vi "Calibrate.vi"(8 "error in (no error)":errorcluster, 11 "Message Queue":refnum<queue>) -> (0 "error out":errorcluster)   [LabVIEW 2020, in "plugin_flodx_pressure.lvlib" / "plugin.lvlib"]
doc: "UI which prompts the user to calibrate the device, in two-point and three-point modes."
uses:
  plugin.lvlib
  <userlib>/RxnRover/PluginCore/src/support/Message Queue/Message Cluster.ctl
  <userlib>/RxnRover/PluginCore/src/support/Message Queue/Message Queue.lvlib
panel:
  in  "Set Ambient Pressure":bool
  in  "Set Ambient Pressure":sgl
  in  "Units":string(combo)
  in  "SHUTDOWN":bool
  in  "Calibrate Button":bool
  # "Device Options"
  # "These are the device options for\nthe FloDx Pressure Sensor. You can\nset the units the device returns,\n(kPa,PSI,BAR) as well as set the\nambient pressure of the device."
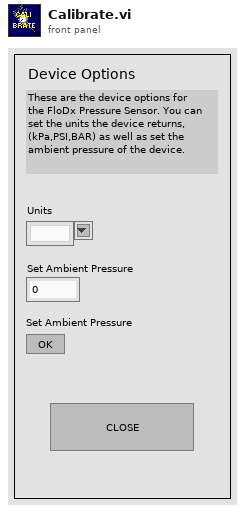
[diagram p1: front panel]
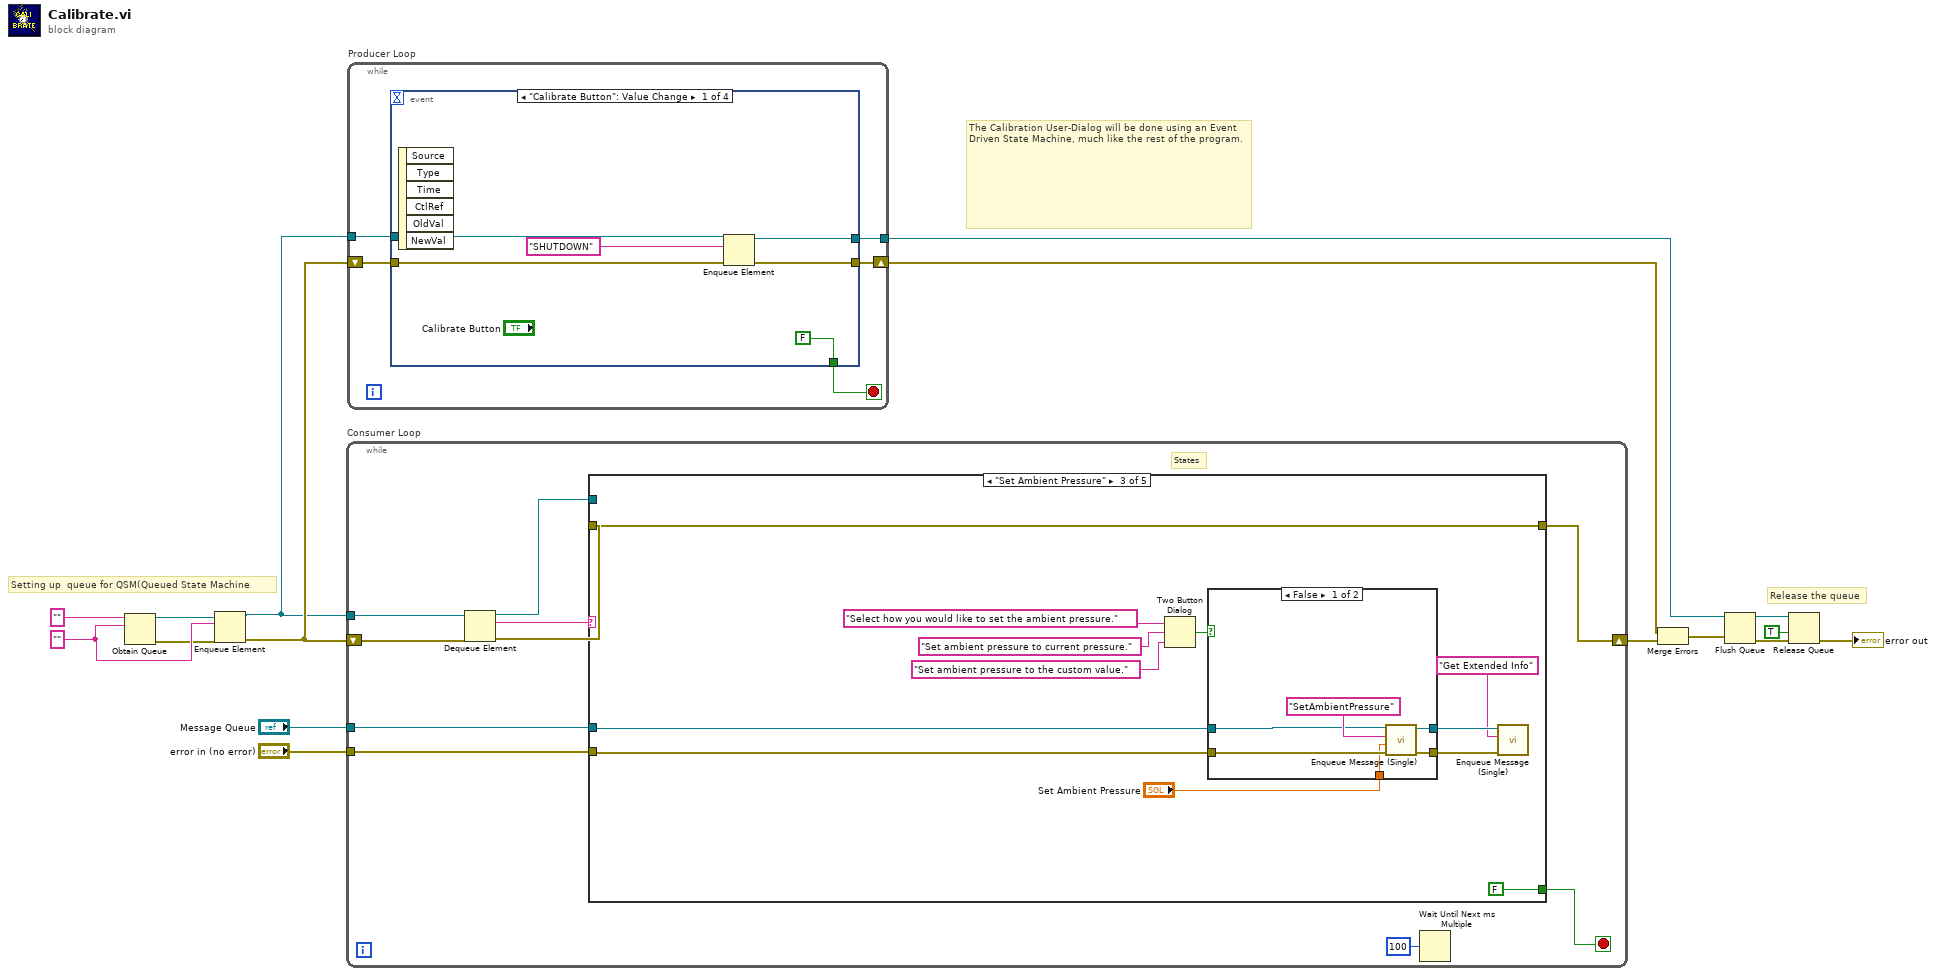
[diagram p0: block diagram]
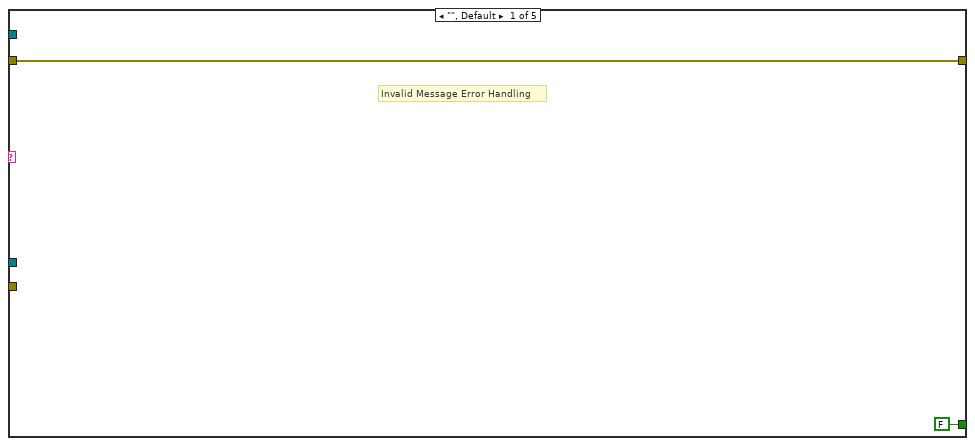
[diagram p2: hidden frame]
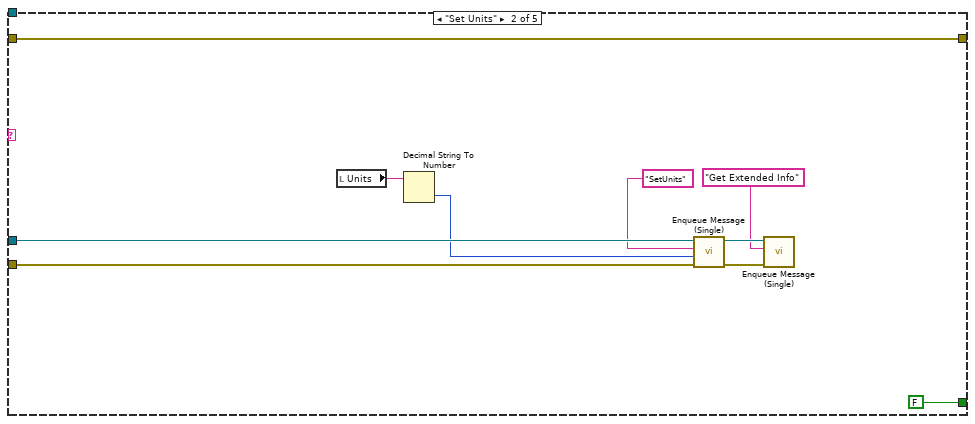
[diagram p3: hidden frame]
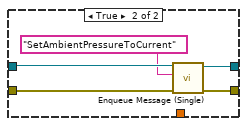
[diagram p4: hidden frame]
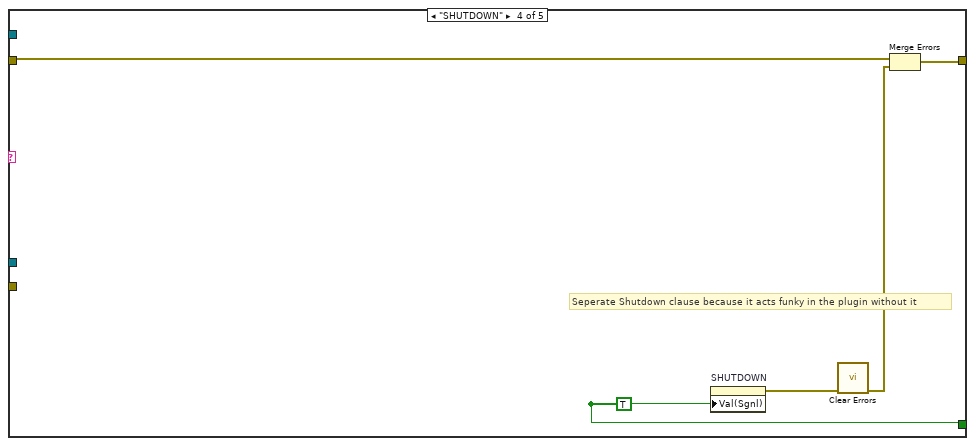
[diagram p5: hidden frame]
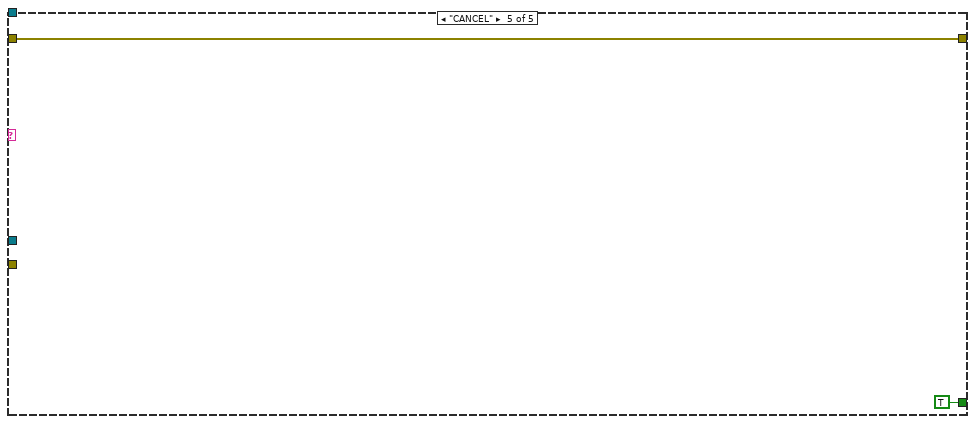
[diagram p6: hidden frame]
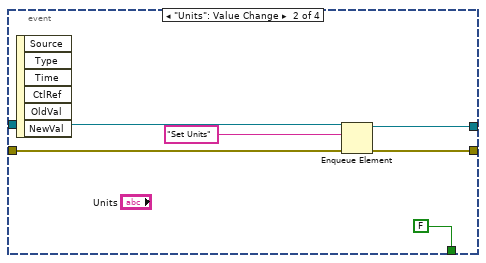
[diagram p7: hidden frame]
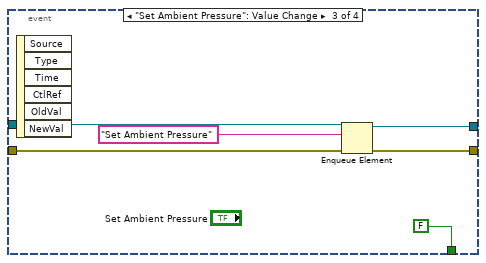
[diagram p8: hidden frame]
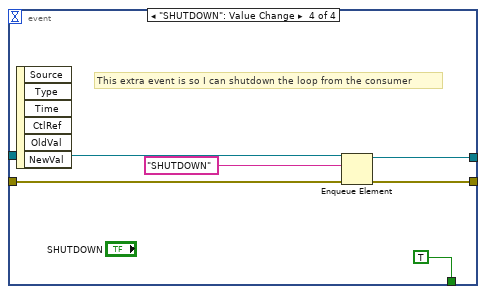
[diagram p9: hidden frame]
diagram:
  w15 = ""
  # "The Calibration User-Dialog will be done using an Event Driven State Machine, much like the rest of the program."
  # "Release the queue"
  # "Setting up  queue for QSM(Queued State Machine"
  n1 = Obtain Queue(name (unnamed)="", element data type=w15) -> (queue out=w14:refnum<queue>, error out=w13:errorcluster)  [unwired: 3 in, 1 out]
  n2 = Enqueue Element(queue=w14, element=w15, error in (no error)=w13) -> (queue out=w1:refnum<queue>, error out=w12:errorcluster)  [unwired: 1 in, 1 out]
  n3 = while "Consumer Loop" {
    tunnel: w1 -> [w26]
    tunnel: "Message Queue" -> [w21]
    tunnel: "error in (no error)" -> [w20]
    shift-right: [w18] -> w9
    shift-left: w12 -> [w17]
    stop <- w22 stop-if-true
    # "States"
    n4 = Dequeue Element(queue=w26, error in (no error)=w17) -> (queue out=w24:refnum<queue>, element=w25:string, error out=w23:errorcluster)  [unwired: 1 in, 1 out]
    n5 = case shown="\"Set Ambient Pressure\"" w25 {
      tunnel: w24 -> [_ _ _ _ _]
      tunnel: w23 -> [w27 w30 w42 w65 w67]
      tunnel: [FALSE ("T button?") FALSE ("T button?") FALSE ("T button?") w62 TRUE ("T button?")] -> w22
      tunnel: w21 -> [_ w37 w44 _ _]
      tunnel: w20 -> [_ w36 w45 _ _]
      tunnel: [w27 w30 w42 w66 w67] -> w18
      frame "", Default {
        # "Invalid Message Error Handling"
      }
      frame "Set Units" {
        n6 = local read "Units"() -> (w29:string)
        n7 = Decimal String To Number(string=w29) -> (number=w34:i32)  [unwired: 2 in, 1 out]
        n8 = call <userlib>:"Enqueue Message (Single).vi"("error in (no error)"=w36, "Message Data"=w34, "Message"="SetUnits", "Message Queue"=w37) -> ("error out"=w32:errorcluster, "dup Message Queue"=w33:refnum<queue>)  [unwired: 6 in]
        n9 = call <userlib>:"Enqueue Message (Single).vi"("error in (no error)"=w32, "Message"="Get Extended Info", "Message Queue"=w33) -> ()  [unwired: 7 in, 2 out]
      }
      frame "Set Ambient Pressure" {
        n10 = Two Button Dialog(message="Select how you would like to set the ambient pressure.", 1:"Set ambient pressure to the custom value." ("F button name (\"Cancel\")"), 2:"Set ambient pressure to current pressure." ("T button name (\"OK\")")) -> (T button?=w48:bool)
        n11 = case shown="False" w48 {
          tunnel: w45 -> [w54 w61]
          tunnel: w44 -> [w55 w60]
          tunnel: "Set Ambient Pressure" -> [w53 _]
          tunnel: [w51 w58] -> w41
          tunnel: [w52 w57] -> w40
          frame False {
            n12 = call <userlib>:"Enqueue Message (Single).vi"("error in (no error)"=w54, "Message Data"=w53, "Message"="SetAmbientPressure", "Message Queue"=w55) -> ("error out"=w51:errorcluster, "dup Message Queue"=w52:refnum<queue>)  [unwired: 6 in]
          }
          frame True {
            n13 = call <userlib>:"Enqueue Message (Single).vi"("error in (no error)"=w61, "Message"="SetAmbientPressureToCurrent", "Message Queue"=w60) -> ("error out"=w58:errorcluster, "dup Message Queue"=w57:refnum<queue>)  [unwired: 7 in]
          }
        }
        n14 = call <userlib>:"Enqueue Message (Single).vi"("error in (no error)"=w41, "Message"="Get Extended Info", "Message Queue"=w40) -> ()  [unwired: 7 in, 2 out]
      }
      frame "SHUTDOWN" {
        w62 = TRUE
        # "Seperate Shutdown clause because it acts funky in the plugin without it"
        n15 = property on="SHUTDOWN" class="Bool (strict)"("Val(Sgnl)"=w62) -> (error out=w63:errorcluster)  [unwired: 2 in, 1 out]
        n16 = call <vilib>:"Clear Errors.vi"("error in (no error)"=w63) -> ("error out"=w64:errorcluster)  [unwired: 5 in, 1 out]
        n17 = Merge Errors(w65, w64) -> (w66:errorcluster)
      }
      frame "CANCEL" {
      }
    }
    n18 = Wait Until Next ms Multiple(millisecond multiple=u32 100) -> ()  [unwired: 1 out]
  }
  n19 = while "Producer Loop" {
    tunnel: w1 -> [w72]
    shift-right: [w70] -> w8
    shift-left: w12 -> [w73]
    tunnel: [w69] -> w6
    stop <- w71 stop-if-true
    n20 = event shown="[0] \"Calibrate Button\": Value Change" {
      selector: _ -> [_ _ _ _]
      dyn-events: _ -> [_ _ _ _]
      timeout: _ -> [_ _ _ _]
      tunnel: w73 -> [w79 w85 w91 w97]
      tunnel: w72 -> [w78 w84 w90 w96]
      tunnel: [w77 w83 w89 w95] -> w69
      tunnel: [FALSE FALSE FALSE TRUE] -> w71
      tunnel: [w74 w80 w86 w92] -> w70
      event "Calibrate Button": Value Change {
        n21 = event-data() -> ()  [unwired: 1 in, 6 out]
        n22 = Enqueue Element(queue=w78, element="SHUTDOWN", error in (no error)=w79) -> (queue out=w77:refnum<queue>, error out=w74:errorcluster)  [unwired: 1 in, 1 out]
      }
      event "Units": Value Change {
        n23 = event-data() -> ()  [unwired: 1 in, 6 out]
        n24 = Enqueue Element(queue=w84, element="Set Units", error in (no error)=w85) -> (queue out=w83:refnum<queue>, error out=w80:errorcluster)  [unwired: 1 in, 1 out]
      }
      event "Set Ambient Pressure": Value Change {
        n25 = event-data() -> ()  [unwired: 1 in, 6 out]
        n26 = Enqueue Element(queue=w90, element="Set Ambient Pressure", error in (no error)=w91) -> (queue out=w89:refnum<queue>, error out=w86:errorcluster)  [unwired: 1 in, 1 out]
      }
      event "SHUTDOWN": Value Change {
        # "This extra event is so I can shutdown the loop from the consumer"
        n27 = event-data() -> ()  [unwired: 1 in, 6 out]
        n28 = Enqueue Element(queue=w96, element="SHUTDOWN", error in (no error)=w97) -> (queue out=w95:refnum<queue>, error out=w92:errorcluster)  [unwired: 1 in, 1 out]
      }
    }
  }
  n29 = Merge Errors(w8, w9) -> (w4:errorcluster)
  n30 = Flush Queue(queue=w6, error in (no error)=w4) -> (queue out=w5:refnum<queue>, error out=w3:errorcluster)  [unwired: 1 out]
  n31 = Release Queue(queue=w5, force destroy? (F)=TRUE, error in (no error)=w3) -> (error out=→"error out":errorcluster)  [unwired: 2 out]
